vi "LSMcontroller_v60_PIzstage.vi"() -> ()   [LabVIEW 2015] (continued)
                                n1732 = Unbundle By Name(w4426) -> ("srate"=w4423:sgl, "Pel"=w4425:sgl)
                                n1733 = To Double Precision Float(number=w4423) -> (double precision float=w4421:dbl)
                                n1734 = To Double Precision Float(number=w4423) -> (double precision float=w4422:dbl)
                                n1735 = To Double Precision Float(number=w4425) -> (double precision float=w4417:dbl)
                                n1736 = Divide(x=w4422, y=w4417) -> (x/y=w4424:dbl)
                                n1737 = Index Array(array=w4434, index=0) -> (element=w4433:T19)
                                n1738 = Divide(x=1.0 ("Digital DC (%)"), y=w4417) -> (x/y=w4419:dbl)
                                n1739 = Multiply(x=100.0, y=w4419) -> (x*y=w4416:dbl)
                                n1740 = Bundle By Name(cluster=w4433, "Digital DC (%)"=w4416, "Digital phase"=w4428, "Digital Freq (Hz)"=w4424, "Sampling frequency (Hz)"=w4421, "Digital time offset (s)"=w4428, "padding value"=0.0, "matlab wave file"=path "LT", "DOtab"=0.0) -> (w4431:T19)
                                n1741 = Build Array(w4431) -> (w4430:T18)
                                n1742 = call "waveformparamsv2.vi"("command"="add DO", "add DO"=w4430) -> ()  [unwired: 3 in, 3 out]
                                }
                                frame 2 {
                                n1743 = call "waveformparamsv2.vi"("command"="get") -> ("Params out"=w4443:T15)  [unwired: 4 in, 2 out]
                                n1744 = in-place {
                                in-place-border: w4441 -> [w4447]
                                in-place-border: [w4446] -> w4440
                                n1745 = in-place-cluster #30(w4443) -> ("DO parameters"=w4449:T18)
                                n1746 = Delete From Array(array=w4449, length=1, index=w4447) -> (deleted portion=w4446:T18, array with subset deleted=w4448:T18)
                                n1747 = in-place-cluster #30("DO parameters"=w4448) -> (w4442:T15)
                                }
                                n1748 = call "waveformparamsv2.vi"("command"="set", "Params in"=w4442) -> ()  [unwired: 3 in, 3 out]
                                }
                                frame 3, Default {
                                }
                                frame 0 {
                                n1749 = local read "Measurement"() -> (w4455:T4)
                                n1750 = To Unsigned Long Integer(number=w4455) -> (unsigned 32bit integer=w4454:u32)
                                n1751 = case shown="5..7" w4454 {
                                tunnel: w4453 -> [_ w4457]
                                tunnel: [_ w4456] -> w4452
                                frame 0..4, Default {
                                }
                                frame 5..7 {
                                n1752 = stacked-sequence {
                                tunnel: w4457 -> [w4459 w4468]
                                tunnel: [w4458 _] -> w4456
                                frame #0 {
                                n1753 = call "waveformparamsv2.vi"("command"="get") -> ("Params out"=w4461:T15)  [unwired: 4 in, 2 out]
                                n1754 = Unbundle By Name(w4461) -> ("DO parameters"=w4462:T18)
                                n1755 = Index Array(array=w4462, index=w4459) -> (element=w4458:T19)
                                }
                                frame #1 {
                                w4476 = 0.0 ("padding value")
                                n1756 = call "2pparameters.vi"("command"="get") -> ("params out"=w4474:T11)  [unwired: 1 in]
                                n1757 = Unbundle By Name(w4474) -> ("srate"=w4472:sgl, "Pel"=w4473:sgl)
                                n1758 = To Double Precision Float(number=w4472) -> (double precision float=w4470:dbl)
                                n1759 = To Double Precision Float(number=w4472) -> (double precision float=w4471:dbl)
                                n1760 = To Double Precision Float(number=w4473) -> (double precision float=w4466:dbl)
                                n1761 = Divide(x=1.0 ("Digital DC (%)"), y=w4466) -> (x/y=w4465:dbl)
                                n1762 = Multiply(x=100.0, y=w4465) -> (x*y=w4464:dbl)
                                n1763 = Divide(x=w4471, y=w4466) -> (x/y=w4469:dbl)
                                n1764 = call "replace DO wf param.vi"("Digital Freq (Hz)"=w4469, "Digital DC (%)"=w4464, "Digital phase"=w4476, "Sampling frequency (Hz)"=w4470, "Digital time offset (s)"=w4476, "index of DO wave"=w4468, "padding value"=w4476, "matlab wave file"=path "LT" ("matlab wave number")) -> ()  [unwired: 3 in]
                                }
                                }
                                }
                                }
                                n1765 = Build Array(w4452) -> (w4451:T18)
                                }
                                }
                                }
                                frame #9 {
                                n1766 = Build Array(w4481, w4480) -> (w4483:bool[])
                                n1767 = Boolean Array To Number(Boolean array=w4483) -> (number=w4482:u32)
                                n1768 = case shown="0" w4482 {
                                tunnel: w4479 -> [_ w4535 _ w4539]
                                tunnel: [_ w4530 _ w4536] -> w4478
                                frame 1 {
                                n1769 = call "2pparameters.vi"("command"="get") -> ("params out"=w4490:T11)  [unwired: 1 in]
                                n1770 = Unbundle By Name(w4490) -> ("wavdet"=w4491:bool, "Pel"=w4493:sgl, "refwfsize"=w4494:dbl, "Pel"=w4492:sgl)
                                n1771 = call "waveformsDObuffer.vi"("command"="get") -> ("DO wf out"=w4486:digitalwaveform[])  [unwired: 1 in]
                                n1772 = case shown="True" w4491 {
                                tunnel: [w4498 w4511] -> w4488
                                tunnel: w4492 -> [w4507 w4526]
                                tunnel: w4493 -> [w4497 w4517]
                                tunnel: w4494 -> [_ w4523]
                                frame False {
                                w4501 = u16 0 items=["unsigned binary", "offset binary", "2's complement"] ("data format (offset binary)")
                                n1773 = Initialize Array(sgl 0.0, w4497) -> (w4504:sgl[])
                                n1774 = Replace Array Subset(array=w4504, new element=sgl 1.0, index=0) -> (w4502:sgl[])
                                n1775 = Reciprocal(x=w4507) -> (1/x=w4508:sgl)
                                n1776 = Bundle By Name("Y"=w4502, "dt"=w4508) -> (w4499:waveform(sgl))  [unwired: 1 in]
                                n1777 = call-poly <vilib>:"Analog to Digital.vi"("data format (offset binary)"=w4501, "compress digital (T)"=TRUE, "full-scale range (pk-pk)"=1.0, "resolution (16 bit)"=1, "analog waveform"=w4499) -> ("digital waveform"=w4498:digitalwaveform)  [unwired: 3 in, 3 out]
                                }
                                frame True {
                                w4514 = u16 0 items=["unsigned binary", "offset binary", "2's complement"] ("data format (offset binary)")
                                n1778 = To Double Precision Float(number=w4517) -> (double precision float=w4524:dbl)
                                n1779 = Initialize Array(sgl 0.0, w4517) -> (w4519:sgl[])
                                n1780 = Divide(x=w4523, y=w4524) -> (x/y=w4521:dbl)
                                n1781 = Round Toward +Infinity(x=w4521) -> (ceil(x): smallest int >= x=w4522:dbl)
                                n1782 = Replace Array Subset(array=w4519, new element=sgl 1.0, index=0) -> (w4516:sgl[])
                                n1783 = for {
                                N: w4522 -> [_]
                                tunnel: w4516 -> [w4528]
                                tunnel: [w4528] -> w4525 mode=concatenating
                                }
                                n1784 = Reciprocal(x=w4526) -> (1/x=w4527:sgl)
                                n1785 = Bundle By Name("Y"=w4525, "dt"=w4527) -> (w4512:waveform(sgl))  [unwired: 1 in]
                                n1786 = call-poly <vilib>:"Analog to Digital.vi"("data format (offset binary)"=w4514, "compress digital (T)"=TRUE, "full-scale range (pk-pk)"=1.0, "resolution (16 bit)"=1, "analog waveform"=w4512) -> ("digital waveform"=w4511:digitalwaveform)  [unwired: 3 in, 3 out]
                                }
                                }
                                n1787 = Build Array (concatenate)(w4486, w4488) -> (w4484:digitalwaveform[])
                                n1788 = call "waveformsDObuffer.vi"("DO wf in"=w4484, "command"="set") -> ()  [unwired: 1 out]
                                }
                                frame 2 {
                                n1789 = call "waveformsDObuffer.vi"("command"="get") -> ("DO wf out"=w4532:digitalwaveform[])  [unwired: 1 in]
                                n1790 = Delete From Array(array=w4532, length=1, index=w4535) -> (deleted portion=w4530:digitalwaveform[], array with subset deleted=w4529:digitalwaveform[])
                                n1791 = call "waveformsDObuffer.vi"("DO wf in"=w4529, "command"="set") -> ()  [unwired: 1 out]
                                }
                                frame 3, Default {
                                }
                                frame 0 {
                                n1792 = local read "Measurement"() -> (w4538:T4)
                                n1793 = To Unsigned Long Integer(number=w4538) -> (unsigned 32bit integer=w4537:u32)
                                n1794 = case shown="5..7" w4537 {
                                tunnel: w4539 -> [_ w4542]
                                tunnel: [_ w4541] -> w4536
                                frame 0..4, Default {
                                }
                                frame 5..7 {
                                n1795 = call "2pparameters.vi"("command"="get") -> ("params out"=w4549:T11)  [unwired: 1 in]
                                n1796 = Unbundle By Name(w4549) -> ("wavdet"=w4550:bool, "Pel"=w4552:sgl, "refwfsize"=w4553:dbl, "srateAODO"=w4551:sgl)
                                n1797 = call "waveformsDObuffer.vi"("command"="get") -> ("DO wf out"=w4543:digitalwaveform[])  [unwired: 1 in]
                                n1798 = Index Array(array=w4543, index=w4542) -> (element=w4544:digitalwaveform)
                                n1799 = case shown="True" w4550 {
                                tunnel: [w4557 w4570] -> w4547
                                tunnel: w4551 -> [w4566 w4585]
                                tunnel: w4552 -> [w4556 w4576]
                                tunnel: w4553 -> [_ w4582]
                                frame False {
                                w4560 = u16 0 items=["unsigned binary", "offset binary", "2's complement"] ("data format (offset binary)")
                                n1800 = Initialize Array(sgl 0.0, w4556) -> (w4563:sgl[])
                                n1801 = Replace Array Subset(array=w4563, new element=sgl 1.0, index=0) -> (w4561:sgl[])
                                n1802 = Reciprocal(x=w4566) -> (1/x=w4567:sgl)
                                n1803 = Bundle By Name("Y"=w4561, "dt"=w4567) -> (w4558:waveform(sgl))  [unwired: 1 in]
                                n1804 = call-poly <vilib>:"Analog to Digital.vi"("data format (offset binary)"=w4560, "compress digital (T)"=TRUE, "full-scale range (pk-pk)"=1.0, "resolution (16 bit)"=1, "analog waveform"=w4558) -> ("digital waveform"=w4557:digitalwaveform)  [unwired: 3 in, 3 out]
                                }
                                frame True {
                                w4573 = u16 0 items=["unsigned binary", "offset binary", "2's complement"] ("data format (offset binary)")
                                n1805 = To Double Precision Float(number=w4576) -> (double precision float=w4583:dbl)
                                n1806 = Initialize Array(sgl 0.0, w4576) -> (w4578:sgl[])
                                n1807 = Divide(x=w4582, y=w4583) -> (x/y=w4580:dbl)
                                n1808 = Round Toward +Infinity(x=w4580) -> (ceil(x): smallest int >= x=w4581:dbl)
                                n1809 = Replace Array Subset(array=w4578, new element=sgl 1.0, index=0) -> (w4575:sgl[])
                                n1810 = for {
                                N: w4581 -> [_]
                                tunnel: w4575 -> [w4587]
                                tunnel: [w4587] -> w4584 mode=concatenating
                                }
                                n1811 = Reciprocal(x=w4585) -> (1/x=w4586:sgl)
                                n1812 = Bundle By Name("Y"=w4584, "dt"=w4586) -> (w4571:waveform(sgl))  [unwired: 1 in]
                                n1813 = call-poly <vilib>:"Analog to Digital.vi"("data format (offset binary)"=w4573, "compress digital (T)"=TRUE, "full-scale range (pk-pk)"=1.0, "resolution (16 bit)"=1, "analog waveform"=w4571) -> ("digital waveform"=w4570:digitalwaveform)  [unwired: 3 in, 3 out]
                                }
                                }
                                n1814 = Build Array(w4544) -> (w4541:digitalwaveform[])
                                n1815 = Replace Array Subset(array=w4543, new element=w4547, index=w4542) -> (w4540:digitalwaveform[])
                                n1816 = call "waveformsDObuffer.vi"("DO wf in"=w4540, "command"="set") -> ()  [unwired: 1 out]
                                }
                                }
                                }
                                }
                                }
                                frame #10 {
                                n1817 = local read "Meastab"() -> (w4601:enum32{"X-Y Image", "Linescan", "Timetrace"})
                                n1818 = property on="refwf" class="Ring (strict)"() -> ("RingText.Text"=w4598:string)  [unwired: 2 in, 2 out]
                                n1819 = case shown="\"Timetrace\"" w4601 {
                                tunnel: [w4603 w4604] -> w4602
                                frame "X-Y Image", Default {
                                n1820 = local read "Sampling rate"() -> (w4603:dbl)
                                }
                                frame "Timetrace" {
                                n1821 = local read "srateAODOtt"() -> (w4604:dbl)
                                }
                                }
                                n1822 = call "waveformsAObuffer.vi"("command"="get") -> ("AO wf out"=w4591:waveform(dbl)[])  [unwired: 1 in]
                                n1823 = local read "wavdet"() -> (w4599:bool)
                                n1824 = call "waveformsDObuffer.vi"("command"="get") -> ("DO wf out"=w4595:digitalwaveform[])  [unwired: 1 in]
                                n1825 = call "correctwaveformsizetemp.vi"("new sampling frequency (Hz)"=w4602, "start"=TRUE, "reference waveforms to"=w4598, "Analog waveforms in"=w4591, "stop"=FALSE, "Digital waveforms in"=w4595) -> ("analog wf out"=w4597:waveform(dbl)[], "Digital wf out"=w4590:digitalwaveform[], "measpoints"=w4600:i32)
                                n1826 = call "waveformsDObuffer.vi"("DO wf in"=w4590, "command"="set") -> ()  [unwired: 1 out]
                                n1827 = call "waveformsAObuffer.vi"("AO wf in"=w4597, "command"="set") -> ()  [unwired: 1 out]
                                n1828 = case shown="True" w4599 {
                                tunnel: w4600 -> [_ w4607]
                                tunnel: w4590 -> [_ w4605]
                                frame False {
                                }
                                frame True {
                                n1829 = local write "# of frames"(w4607) -> ()
                                n1830 = call "GetNumCamFramesv2.vi"("Digital Waveform Graph"=w4605) -> ("Numeric"=w4606:i32)  [unwired: 10 in]
                                n1831 = local write "Total Camera Frames"(w4606) -> ()
                                }
                                }
                                }
                                }
                              }
                              frame #7 {
                                # "Disabled for conversion to 64 bit"
                                n1832 = disable-structure shown="Disabled" {
                                frame Disabled {
                                n1833 = local read "Measurement"() -> (w4609:T4)
                                n1834 = case shown="\"Lifetime (scan)\"" w4609 {
                                frame "X-Y-t movie", Default {
                                }
                                frame "Lifetime (scan)" {
                                # "total acquisition time"
                                n1835 = call "2pparameters.vi"("command"="get") -> ("params out"=w4617:T11)  [unwired: 1 in]
                                n1836 = Unbundle By Name(w4617) -> ("measpoints"=w4611:i32, "srateAODO"=w4632:sgl)
                                n1837 = Divide(x=w4611, y=w4632) -> (x/y=w4610:sgl)
                                n1838 = local read "min phot"() -> (w4627:u32)
                                n1839 = local read "expected c/s"() -> (w4628:dbl)
                                n1840 = Multiply(x=w4610, y=1000.0) -> (x*y=w4620:dbl)
                                n1841 = local read "Ch1 ZeroX"() -> (w4625:i32)
                                n1842 = local read "truncate"() -> (w4626:u32)
                                n1843 = To Long Integer(number=w4620) -> (32bit integer=w4629:i32)
                                n1844 = To Long Integer(number=w4628) -> (32bit integer=w4630:i32)
                                n1845 = local read "Number of Bins"() -> (w4621:u32)
                                n1846 = local read "Ch1 Level"() -> (w4623:i32)
                                n1847 = local read "Ch0 ZeroX"() -> (w4624:i32)
                                n1848 = local write "Acquisition time"(w4629) -> ()
                                n1849 = local read "Ch0 Level"() -> (w4622:i32)
                                n1850 = call "lifetimeparameters.vi"("command"="get") -> ("Params out"=w4615:T20)  [unwired: 1 in]
                                n1851 = Add(x=100, y=w4629) -> (x+y=w4619:i32)
                                n1852 = Bundle By Name(cluster=w4615, "acq time"=w4619, "acq rate"=w4630, "# bins"=w4621, "Ch0 Level"=w4622, "Ch1 Level"=w4623, "Ch0 ZeroX"=w4624, "Ch1 ZeroX"=w4625, "min photons"=w4627, "truncate"=w4626) -> (w4614:T20)
                                n1853 = local write "Acquisition rate"(w4630) -> ()
                                n1854 = call "lifetimeparameters.vi"("Params in"=w4614, "command"="set") -> ()  [unwired: 1 out]
                                }
                                }
                                }
                                frame Enabled {
                                }
                                }
                                n1855 = local write "64bit disabled"(TRUE ("64bit disabled")) -> ()
                              }
                              frame #8 {
                                n1856 = call "2pparameters.vi"("command"="get") -> ("params out"=w4643:T11)  [unwired: 1 in]
                                n1857 = Unbundle By Name(w4643) -> ("refreshbuffer"=w4641:i32, "srate"=w4642:sgl)
                                n1858 = local read "wavdet"() -> (w4633:bool)
                                n1859 = To Double Precision Float(number=w4642) -> (double precision float=w4645:dbl)
                                n1860 = To Double Precision Float(number=w4641) -> (double precision float=w4636:dbl)
                                n1861 = case shown="False" w4633 {
                                tunnel: [w4650 w4651] -> w4635
                                frame False {
                                w4650 = 10123 items=["Finite Samples"=10178, "Continuous Samples"=10123, "Hardware Timed Single Point"=12522] ("sample mode")
                                }
                                frame True {
                                w4651 = 10123 items=["Finite Samples"=10178, "Continuous Samples"=10123, "Hardware Timed Single Point"=12522] ("sample mode")
                                }
                                }
                                n1862 = Divide(x=w4636, y=w4645) -> (x/y=w4649:dbl)
                                n1863 = Multiply(x=w4649, y=2.0) -> (x*y=w4646:dbl)
                                n1864 = Max & Min(x=w4646, y=10.0) -> (max(x,y)=w4637:dbl)  [unwired: 1 out]
                                n1865 = call "2pparameters.vi"("command"="get") -> ("params out"=w4640:T11)  [unwired: 1 in]
                                n1866 = Bundle By Name(cluster=w4640, "timeout"=w4637, "sample mode"=w4635) -> (w4638:T11)
                                n1867 = call "2pparameters.vi"("Params in"=w4638, "command"="set") -> ()  [unwired: 1 out]
                              }
                            }
                          }
                          frame #1 {
                            # "Disabled for conversion to 64 bit"
                            n1868 = call "prepAO_img.vi"() -> ("Terminal Name with Device Prefix"=w4653:tag)
                            n1869 = call "prepDO_img.vi"() -> ()  [unwired: 2 in]
                            n1870 = call "prepAI_img.vi"("triggersource"=w4653) -> ()  [unwired: 2 in]
                            n1871 = call "prepCI_img.vi"("ArmStart.DigEdge.Src"=w4653) -> ()  [unwired: 1 in]
                            n1872 = disable-structure shown="Disabled" {
                              frame Disabled {
                                n1873 = local read "Measurement"() -> (w4654:T4)
                                n1874 = case shown="\"Lifetime (contour)\"" w4654 {
                                frame "X-Y-t movie", Default {
                                }
                                frame "Lifetime (contour)" {
                                n1875 = stacked-sequence {
                                frame #0 {
                                n1876 = call "PH-temp.vi"("String"="clear" ("command")) -> ()  [unwired: 2 in, 2 out]
                                n1877 = call "PH-temp-raw.vi"("command"="empty") -> ()  [unwired: 1 in, 1 out]
                                }
                                frame #1 {
                                n1878 = call "calib.vi"() -> ()  [unwired: 1 in]
                                }
                                frame #2 {
                                n1879 = call "setup.vi"() -> ()  [unwired: 1 in]
                                }
                                }
                                }
                                }
                              }
                              frame Enabled {
                              }
                            }
                            n1880 = local write "64bit disabled"(TRUE ("64bit disabled")) -> ()
                          }
                          frame #2 {
                            n1881 = local read "save\ndata"() -> (w4657:bool)
                            n1882 = case shown="True" w4657 {
                              tunnel: w4658 -> [_ w4662]
                              frame False {
                              }
                              frame True {
                                n1883 = local read "filename prefix"() -> (w4660:string)
                                n1884 = local read "data dir"() -> (w4661:path)
                                n1885 = call "preparebinaryfiles.vi"("filename prefix"=w4660, "data dir"=w4661, "timestamp"=w4662) -> ("full-filename"=w4659:string)  [unwired: 1 in]
                                n1886 = local write "full-filename"(w4659) -> ()
                              }
                            }
                            n1887 = call "preptempbuffers_tt.vi"() -> ()  [unwired: 12 in]
                          }
                          frame #3 {
                            n1888 = local read "wavdet"() -> (w4663:bool)
                            n1889 = case shown="False" w4663 {
                              frame False {
                                n1890 = disable-structure shown="Disabled" {
                                frame Disabled {
                                n1891 = call "2pparameters.vi"("command"="get") -> ("params out"=w4665:T11)  [unwired: 1 in]
                                n1892 = Unbundle By Name(w4665) -> ("autoshutter"=w4666:bool)
                                n1893 = case shown="True" w4666 {
                                frame False {
                                }
                                frame True {
                                n1894 = call "shuttercontrol.vi"("command"="open") -> ()  [unwired: 1 in, 1 out]
                                }
                                }
                                }
                                frame Enabled {
                                }
                                }
                              }
                              frame True {
                              }
                            }
                          }
                          frame #4 {
                            n1895 = flat-sequence {
                              frame #0 {
                                # "Disabled for conversion to 64 bit"
                                n1896 = disable-structure shown="Disabled" {
                                frame Disabled {
                                n1897 = local read "Measurement"() -> (w4669:T4)
                                n1898 = case shown="\"Lifetime (contour)\"" w4669 {
                                frame "X-Y-t movie", Default {
                                }
                                frame "Lifetime (contour)" {
                                n1899 = call "runLT_img.vi"() -> ()  [unwired: 1 in]
                                }
                                }
                                }
                                frame Enabled {
                                }
                                }
                                n1900 = local write "64bit disabled"(TRUE ("64bit disabled")) -> ()
                              }
                              frame #1 {
                                n1901 = call "runAI_img.vi"() -> ()  [unwired: 12 in]
                                n1902 = call "runCI.vi"() -> ()  [unwired: 12 in]
                                n1903 = call "runDO_img.vi"() -> ()  [unwired: 12 in]
                              }
                              frame #2 {
                                n1904 = call "runAO_img.vi"() -> ()  [unwired: 12 in]
                              }
                            }
                          }
                          frame #5 {
                            # "Disabled for conversion to 64 bit"
                            n1905 = disable-structure shown="Disabled" {
                              disable-tunnel: w4671 -> [w4672 _]
                              frame Disabled {
                                w4675 = u16 0 items=["Stream to disk", "Post process", "real time process"] ("Ring")
                                n1906 = local read "T3R Data processing"() -> (w4674:u16)
                                n1907 = Equal?(x=w4674, y=w4675) -> (x = y?=w4673:bool)
                                n1908 = local read "save\ndata"() -> (w4677:bool)
                                n1909 = local read "Measurement"() -> (w4678:T4)
                                n1910 = And(x=w4677, y=w4673) -> (x .and. y?=w4676:bool)
                                n1911 = case shown="\"Lifetime (contour)\"" w4678 {
                                tunnel: w4672 -> [_ w4682]
                                tunnel: w4676 -> [_ w4680]
                                frame "X-Y-t movie", Default {
                                }
                                frame "Lifetime (contour)" {
                                n1912 = case shown="True" w4680 {
                                selector: w4680 -> [w4683 w4688]
                                tunnel: w4682 -> [_ w4686]
                                tunnel: [path "" ("appended path") w4689] -> w4681
                                tunnel: [w4683 w4688] -> w4679
                                frame False {
                                }
                                frame True {
                                n1913 = local read "filename prefix"() -> (w4687:string)
                                n1914 = local read "data dir"() -> (w4690:path)
                                n1915 = call "generatedatafilename.vi"("timestamp"=w4686, "filename prefix in"=w4687) -> ("full-filename"=w4685:string)
                                n1916 = Concatenate Strings(w4685, ".lvpt3contour" ("string")) -> (w4692:string)
                                n1917 = Build Path(base path=w4690, name or relative path=w4692) -> (appended path=w4689:path)
                                }
                                }
                                n1918 = call "collectLT_res_v1.vi"("stream?"=w4679, "data file"=w4681) -> ()  [unwired: 2 out]
                                }
                                }
                              }
                              frame Enabled {
                              }
                            }
                            n1919 = while {
                              i -> [w4695]
                              stop <- w4693 stop-if-true
                              n1920 = local read "Stop"() -> (w4703:bool)
                              n1921 = local read "Exit"() -> (w4702:bool)
                              n1922 = Increment(x=w4695) -> (x+1=w4694:i32)
                              n1923 = local write "points recorded"(w4694) -> ()
                              n1924 = Or(x=w4703, y=w4702) -> (x .or. y?=w4701:bool)
                              n1925 = case shown="False" w4701 {
                                frame False {
                                n1926 = stacked-sequence {
                                frame #0 {
                                n1927 = call "collectAI_tt_V2.vi"() -> ()  [unwired: 4 in]
                                n1928 = call "collectCI_tt.vi"() -> ("size(s)"=w4710:i32)  [unwired: 3 in]
                                n1929 = local write "scol"(w4710) -> ()
                                }
                                frame #1 {
                                n1930 = local read "Live"() -> (w4711:bool)
                                n1931 = case shown="True" w4711 {
                                frame False {
                                }
                                frame True {
                                n1932 = local read "graph1list"() -> (w4718:u16)
                                n1933 = local read "graph2list"() -> (w4717:u16)
                                n1934 = To Unsigned Word Integer(number=w4718) -> (unsigned 16bit integer=w4716:u16)
                                n1935 = To Unsigned Word Integer(number=w4717) -> (unsigned 16bit integer=w4715:u16)
                                n1936 = call "dattotrace.vi"("graph2list"=w4715, "Current Average"=sgl 1.0, "graph1list"=w4716) -> ("trace2array out"=w4713:sgl[], "trace1array out"=w4724:sgl[])
                                n1937 = local read "bin"() -> (w4725:dbl)
                                n1938 = script code="data=reshape(datain,[bin length(datain)./bin]);\ndataout=mean(data,1);\ndata2=reshape(datain2,[bin length(datain2)./bin]);\ndataout2=mean(data2,1);"("bin"=w4725, "datain"=w4724, "datain2"=w4713) -> ("dataout"=w4723:dbl[], "dataout2"=w4712:dbl[])  [unwired: 1 in, 1 out]
                                n1939 = Array Size(array=w4712) -> (size(s)=w4726:i32)
                                n1940 = Divide(x=w4726, y=2) -> (x/y=w4728:dbl)
                                n1941 = Round To Nearest(number=w4728) -> (nearest integer value=w4730:dbl)
                                n1942 = Array Size(array=w4723) -> (size(s)=w4735:i32)
                                n1943 = Delete From Array(array=w4712, length=w4730, index=0) -> (deleted portion=w4721:dbl[], array with subset deleted=w4722:dbl[])
                                n1944 = Divide(x=w4735, y=2) -> (x/y=w4733:dbl)
                                n1945 = Round To Nearest(number=w4733) -> (nearest integer value=w4731:dbl)
                                n1946 = Delete From Array(array=w4723, length=w4731, index=0) -> (deleted portion=w4720:dbl[], array with subset deleted=w4719:dbl[])
                                n1947 = local write "graph2"(w4719) -> ()
                                n1948 = local write "graph1"(w4720) -> ()
                                n1949 = local write "graph3"(w4721) -> ()
                                n1950 = local write "graph4"(w4722) -> ()
                                }
                                }
                                }
                                frame #2 {
                                n1951 = local read "save\ndata"() -> (w4736:bool)
                                n1952 = case shown="True" w4736 {
                                frame False {
                                }
                                frame True {
                                n1953 = call "savebinaryfiles.vi"() -> ()  [unwired: 1 in]
                                }
                                }
                                }
                                }
                                }
                                frame True {
                                }
                              }
                              n1954 = local read "continuous"() -> (w4698:bool)
                              n1955 = case shown="False" w4698 {
                                tunnel: w4694 -> [w4708 _]
                                tunnel: [w4707 FALSE] -> w4696
                                frame False {
                                n1956 = call "2pparameters.vi"("command"="get") -> ("params out"=w4705:T11)  [unwired: 1 in]
                                n1957 = Unbundle By Name(w4705) -> ("tt_cycles"=w4704:i32)
                                n1958 = Greater Or Equal?(x=w4708, y=w4704) -> (x >= y?=w4707:bool)
                                }
                                frame True {
                                }
                              }
                              n1959 = local read "Stop"() -> (w4700:bool)
                              n1960 = local read "Exit"() -> (w4699:bool)
                              n1961 = Or(x=w4700, y=w4699) -> (x .or. y?=w4697:bool)
                              n1962 = Or(x=w4697, y=w4696) -> (x .or. y?=w4693:bool)
                            }
                            n1963 = local write "64bit disabled"(TRUE ("64bit disabled")) -> ()
                          }
                          frame #6 {
                            # "Disabled for conversion to 64 bit"
                            n1964 = local read "Measurement"() -> (w4739:T4)
                            n1965 = disable-structure shown="Disabled" {
                              disable-tunnel: w4739 -> [w4741 _]
                              disable-tunnel: w4738 -> [w4740 _]
                              frame Disabled {
                                n1966 = case shown="\"Lifetime (contour)\"" w4741 {
                                tunnel: w4740 -> [_ w4742]
                                frame "X-Y-t movie", Default {
                                }
                                frame "Lifetime (contour)" {
                                n1967 = stacked-sequence {
                                tunnel: w4742 -> [_ w4743]
                                frame #0 {
                                n1968 = flat-sequence {
                                frame #0 {
                                n1969 = call "stoperaseLT_img.vi"() -> ()  [unwired: 1 in]
                                }
                                }
                                }
                                frame #1 {
                                w4746 = u16 0 items=["Stream to disk", "Post process", "real time process"] ("Ring")
                                n1970 = local read "T3R Data processing"() -> (w4745:u16)
                                n1971 = local read "save\ndata"() -> (w4748:bool)
                                n1972 = Equal?(x=w4745, y=w4746) -> (x = y?=w4744:bool)
                                n1973 = Not(x=w4744) -> (.not. x?=w4749:bool)
                                n1974 = And(x=w4748, y=w4749) -> (x .and. y?=w4747:bool)
                                n1975 = case shown="True" w4747 {
                                tunnel: w4743 -> [_ w4750]
                                frame False {
                                }
                                frame True {
                                n1976 = local read "filename prefix"() -> (w4751:string)
                                n1977 = local read "data dir"() -> (w4767:path)
                                n1978 = call "2pparameters.vi"("command"="get") -> ("params out"=w4762:T11)  [unwired: 1 in]
                                n1979 = call "generatedatafilename.vi"("timestamp"=w4750, "filename prefix in"=w4751) -> ("full-filename"=w4752:string)
                                n1980 = Unbundle By Name(w4762) -> ("srate"=w4760:sgl, "Pel"=w4759:sgl, "measpoints"=w4757:i32)
                                n1981 = Concatenate Strings(w4752, ".lvpt3contour" ("string")) -> (w4765:string)
                                n1982 = Build Path(base path=w4767, name or relative path=w4765) -> (appended path=w4764:path)
                                n1983 = To Unsigned Long Integer(number=w4760) -> (unsigned 32bit integer=w4761:u32)
                                n1984 = To Unsigned Long Integer(number=w4759) -> (unsigned 32bit integer=w4758:u32)
                                n1985 = To Unsigned Long Integer(number=w4757) -> (unsigned 32bit integer=w4756:u32)
                                n1986 = call "PH-temp-raw.vi"("command"="get") -> ("array out"=w4755:u32[])  [unwired: 1 in]
                                n1987 = Build Array (concatenate)(w4761, w4758, w4756, w4755) -> (w4754:u32[])
                                n1988 = Open/Create/Replace File(file path (use dialog)=w4764, operation (0:open)=T8."replace or create") -> (refnum out=w4771:refnum<file>, error out=w4770:errorcluster)  [unwired: 4 in, 1 out]
                                n1989 = Write to Binary File(file (use dialog)=w4771, data=w4754, error in=w4770, 5:FALSE ("prepend array or string size? (T)")) -> (refnum out=w4768:refnum<file>, error out=w4769:errorcluster)  [unwired: 2 in, 1 out]
                                n1990 = Close File(refnum=w4768, error in=w4769) -> ()  [unwired: 2 out]
                                }
                                }
                                }
                                }
                                }
                                }
                              }
                              frame Enabled {
                              }
                            }
                            n1991 = local write "64bit disabled"(TRUE ("64bit disabled")) -> ()
                          }
                          frame #7 {
                            n1992 = call "reset AO_DO_v3.vi"() -> ()  [unwired: 12 in]
                          }
                          frame #8 {
                            n1993 = stacked-sequence {
                              tunnel: w4787 -> [w4790 _ _ _ _ _]
                              tunnel: w4784 -> [w4789 _ _ _ _ _]
                              tunnel: w4785 -> [w4788 _ _ _ _ _]
                              tunnel: w4786 -> [_ w4839 _ _ _ _]
                              tunnel: w4782 -> [_ w4838 w4893 w4990 _ _]
                              tunnel: w4783 -> [_ w4837 w4892 w4989 _ _]
                              tunnel: w4781 -> [_ _ _ w4988 _ _]
                              tunnel: w4780 -> [_ _ _ w4987 _ _]
                              tunnel: w4779 -> [_ _ w4890 _ _ _]
                              tunnel: w4778 -> [_ _ w4889 _ _ _]
                              tunnel: w4777 -> [_ _ w4887 _ _ _]
                              tunnel: w4776 -> [_ _ w4886 _ _ _]
                              tunnel: w4775 -> [_ _ _ w4985 _ _]
                              tunnel: w4774 -> [_ _ _ w4984 _ _]
                              frame #0 {
                                n1994 = case shown="False" w4790 {
                                tunnel: w4789 -> [_ w4812]
                                tunnel: w4788 -> [_ w4811]
                                frame True {
                                n1995 = stacked-sequence {
                                seq-local: [w4791 _ _] -> [_ w4803 w4808]
                                frame #0 {
                                n1996 = call "configuration.vi"("command"="get") -> ("config out"=w4797:T12)  [unwired: 2 in, 1 out]
                                n1997 = Unbundle By Name(w4797) -> ("Voltage to Xgalvo"=w4794:i32)
                                n1998 = call "2pparameters.vi"("command"="get") -> ("params out"=w4795:T11)  [unwired: 1 in]
                                n1999 = in-place {
                                in-place-border: w4794 -> [w4802]
                                in-place-border: [w4799] -> w4791
                                n2000 = in-place-cluster #31(w4795) -> ("aAO"=w4801:u32[])
                                n2001 = call "remove channel from active arrayv2.vi"("line array in"=w4801, "line to remove"=w4802) -> ("line array out"=w4800:u32[], "index"=w4799:i32)  [unwired: 1 out]
                                n2002 = in-place-cluster #31("aAO"=w4800) -> (w4792:T11)
                                }
                                n2003 = call "2pparameters.vi"("Params in"=w4792, "command"="set") -> ()  [unwired: 1 out]
                                }
                                frame #1 {
                                n2004 = call "waveformparamsv2.vi"("command"="rem AO", "index"=w4803) -> ()  [unwired: 3 in, 3 out]
                                }
                                frame #2 {
                                n2005 = call "waveformsAObuffer.vi"("command"="get") -> ("AO wf out"=w4809:waveform(dbl)[])  [unwired: 1 in]
                                n2006 = Delete From Array(array=w4809, length=1, index=w4808) -> (array with subset deleted=w4805:waveform(dbl)[])  [unwired: 1 out]
                                n2007 = call "waveformsAObuffer.vi"("AO wf in"=w4805, "command"="set") -> ()  [unwired: 1 out]
                                }
                                }
                                }
                                frame False {
                                n2008 = stacked-sequence {
                                seq-local: [w4813 _ _] -> [_ w4821 w4832]
                                tunnel: w4812 -> [_ w4820 _]
                                tunnel: w4811 -> [_ _ w4831]
                                frame #0 {
                                n2009 = call "configuration.vi"("command"="get") -> ("config out"=w4818:T12)  [unwired: 2 in, 1 out]
                                n2010 = Unbundle By Name(w4818) -> ("Voltage to Xgalvo"=w4814:i32)
                                n2011 = call "2pparameters.vi"("command"="get") -> ("params out"=w4817:T11)  [unwired: 1 in]
                                n2012 = Unbundle By Name(w4817) -> ("aAO"=w4815:u32[])
                                n2013 = Search 1D Array(1D array=w4815, element=w4814) -> (index of element=w4813:i32)  [unwired: 1 in]
                                }
                                frame #1 {
                                n2014 = call "waveformparamsv2.vi"("command"="get") -> ("Params out"=w4824:T15)  [unwired: 4 in, 2 out]
                                n2015 = in-place {
                                in-place-border: w4821 -> [w4828]
                                in-place-border: w4820 -> [w4827]
                                n2016 = in-place-cluster #32(w4824) -> ("AO parameters"=w4829:T16)
                                n2017 = in-place {
                                in-place-border: w4827 -> [w4830]
                                n2018 = in-place-array #33(w4829, w4828) -> ()  [unwired: 1 out]
                                n2019 = in-place-array #33(w4830) -> (w4826:T16)  [unwired: 1 out]
                                }
                                n2020 = in-place-cluster #32("AO parameters"=w4826) -> (w4822:T15)
                                }
                                n2021 = call "waveformparamsv2.vi"("command"="set", "Params in"=w4822) -> ()  [unwired: 3 in, 3 out]
                                }
                                frame #2 {
                                n2022 = call "waveformsAObuffer.vi"("command"="get") -> ("AO wf out"=w4835:waveform(dbl)[])  [unwired: 1 in]
                                n2023 = Replace Array Subset(array=w4835, new element=w4831, index=w4832) -> (w4833:waveform(dbl)[])
                                n2024 = call "waveformsAObuffer.vi"("AO wf in"=w4833, "command"="set") -> ()  [unwired: 1 out]
                                }
                                }
                                }
                                }
                              }
                              frame #1 {
                                n2025 = case shown="False" w4839 {
                                tunnel: w4838 -> [_ w4861]
                                tunnel: w4837 -> [_ w4860]
                                frame True {
                                n2026 = stacked-sequence {
                                seq-local: [w4840 _ _] -> [_ w4852 w4857]
                                frame #0 {
                                n2027 = call "configuration.vi"("command"="get") -> ("config out"=w4846:T12)  [unwired: 2 in, 1 out]
                                n2028 = Unbundle By Name(w4846) -> ("Voltage to Ygalvo"=w4843:i32)
                                n2029 = call "2pparameters.vi"("command"="get") -> ("params out"=w4844:T11)  [unwired: 1 in]
                                n2030 = in-place {
                                in-place-border: w4843 -> [w4851]
                                in-place-border: [w4848] -> w4840
                                n2031 = in-place-cluster #34(w4844) -> ("aAO"=w4850:u32[])
                                n2032 = call "remove channel from active arrayv2.vi"("line array in"=w4850, "line to remove"=w4851) -> ("line array out"=w4849:u32[], "index"=w4848:i32)  [unwired: 1 out]
                                n2033 = in-place-cluster #34("aAO"=w4849) -> (w4841:T11)
                                }
                                n2034 = call "2pparameters.vi"("Params in"=w4841, "command"="set") -> ()  [unwired: 1 out]
                                }
                                frame #1 {
                                n2035 = call "waveformparamsv2.vi"("command"="rem AO", "index"=w4852) -> ()  [unwired: 3 in, 3 out]
                                }
                                frame #2 {
                                n2036 = call "waveformsAObuffer.vi"("command"="get") -> ("AO wf out"=w4858:waveform(dbl)[])  [unwired: 1 in]
                                n2037 = Delete From Array(array=w4858, length=1, index=w4857) -> (array with subset deleted=w4854:waveform(dbl)[])  [unwired: 1 out]
                                n2038 = call "waveformsAObuffer.vi"("AO wf in"=w4854, "command"="set") -> ()  [unwired: 1 out]
                                }
                                }
                                }
                                frame False {
                                n2039 = stacked-sequence {
                                seq-local: [w4862 _ _] -> [_ w4870 w4881]
                                tunnel: w4861 -> [_ w4869 _]
                                tunnel: w4860 -> [_ _ w4880]
                                frame #0 {
                                n2040 = call "configuration.vi"("command"="get") -> ("config out"=w4867:T12)  [unwired: 2 in, 1 out]
                                n2041 = Unbundle By Name(w4867) -> ("Voltage to Ygalvo"=w4863:i32)
                                n2042 = call "2pparameters.vi"("command"="get") -> ("params out"=w4866:T11)  [unwired: 1 in]
                                n2043 = Unbundle By Name(w4866) -> ("aAO"=w4864:u32[])
                                n2044 = Search 1D Array(1D array=w4864, element=w4863) -> (index of element=w4862:i32)  [unwired: 1 in]
                                }
                                frame #1 {
                                n2045 = call "waveformparamsv2.vi"("command"="get") -> ("Params out"=w4873:T15)  [unwired: 4 in, 2 out]
                                n2046 = in-place {
                                in-place-border: w4870 -> [w4877]
                                in-place-border: w4869 -> [w4876]
                                n2047 = in-place-cluster #35(w4873) -> ("AO parameters"=w4878:T16)
                                n2048 = in-place {
                                in-place-border: w4876 -> [w4879]
                                n2049 = in-place-array #36(w4878, w4877) -> ()  [unwired: 1 out]
                                n2050 = in-place-array #36(w4879) -> (w4875:T16)  [unwired: 1 out]
                                }
                                n2051 = in-place-cluster #35("AO parameters"=w4875) -> (w4871:T15)
                                }
                                n2052 = call "waveformparamsv2.vi"("command"="set", "Params in"=w4871) -> ()  [unwired: 3 in, 3 out]
                                }
                                frame #2 {
                                n2053 = call "waveformsAObuffer.vi"("command"="get") -> ("AO wf out"=w4884:waveform(dbl)[])  [unwired: 1 in]
                                n2054 = Replace Array Subset(array=w4884, new element=w4880, index=w4881) -> (w4882:waveform(dbl)[])
                                n2055 = call "waveformsAObuffer.vi"("AO wf in"=w4882, "command"="set") -> ()  [unwired: 1 out]
                                }
                                }
                                }
                                }
                              }
                              frame #2 {
                                n2056 = Build Array(w4890, w4889) -> (w4891:bool[])
                                n2057 = Boolean Array To Number(Boolean array=w4891) -> (number=w4888:u32)
                                n2058 = case shown="2" w4888 {
                                tunnel: w4893 -> [_ _ w4936]
                                tunnel: w4892 -> [_ _ w4935]
                                tunnel: w4887 -> [_ w4915 w4934]
                                tunnel: w4886 -> [_ w4914 w4933]
                                frame 1, Default {
                                n2059 = stacked-sequence {
                                seq-local: [w4894 _ _] -> [_ w4906 w4911]
                                frame #0 {
                                n2060 = call "configuration.vi"("command"="get") -> ("config out"=w4900:T12)  [unwired: 2 in, 1 out]
                                n2061 = Unbundle By Name(w4900) -> ("2P shutter"=w4897:i32)
                                n2062 = call "2pparameters.vi"("command"="get") -> ("params out"=w4898:T11)  [unwired: 1 in]
                                n2063 = in-place {
                                in-place-border: w4897 -> [w4905]
                                in-place-border: [w4902] -> w4894
                                n2064 = in-place-cluster #37(w4898) -> ("aDO"=w4904:u32[])
                                n2065 = call "remove channel from active arrayv2.vi"("line array in"=w4904, "line to remove"=w4905) -> ("line array out"=w4903:u32[], "index"=w4902:i32)  [unwired: 1 out]
                                n2066 = in-place-cluster #37("aDO"=w4903) -> (w4895:T11)
                                }
                                n2067 = call "2pparameters.vi"("Params in"=w4895, "command"="set") -> ()  [unwired: 1 out]
                                }
                                frame #1 {
                                n2068 = call "waveformparamsv2.vi"("command"="rem DO", "index"=w4906) -> ()  [unwired: 3 in, 3 out]
                                }
                                frame #2 {
                                n2069 = call "waveformsDObuffer.vi"("command"="get") -> ("DO wf out"=w4912:digitalwaveform[])  [unwired: 1 in]
                                n2070 = Delete From Array(array=w4912, length=1, index=w4911) -> (array with subset deleted=w4908:digitalwaveform[])  [unwired: 1 out]
                                n2071 = call "waveformsDObuffer.vi"("DO wf in"=w4908, "command"="set") -> ()  [unwired: 1 out]
                                }
                                }
                                }
                                frame 2 {
                                n2072 = stacked-sequence {
                                tunnel: w4915 -> [_ w4926 _]
                                tunnel: w4914 -> [_ _ w4928]
                                frame #0 {
                                n2073 = call "configuration.vi"("command"="get") -> ("config out"=w4917:T12)  [unwired: 2 in, 1 out]
                                n2074 = call "2pparameters.vi"("command"="get") -> ("params out"=w4921:T11)  [unwired: 1 in]
                                n2075 = Unbundle By Name(w4917) -> ("2P shutter"=w4916:i32)
                                n2076 = in-place {
                                in-place-border: w4916 -> [w4925]
                                n2077 = in-place-cluster #38(w4921) -> ("aDO"=w4924:u32[])
                                n2078 = call "add channel to active arrayv2.vi"("line array in"=w4924, "line to add"=w4925) -> ("line array out"=w4923:u32[])  [unwired: 2 out]
                                n2079 = in-place-cluster #38("aDO"=w4923) -> (w4919:T11)
                                }
                                n2080 = call "2pparameters.vi"("Params in"=w4919, "command"="set") -> ()  [unwired: 1 out]
                                }
                                frame #1 {
                                n2081 = call "waveformparamsv2.vi"("command"="add DO", "add DO"=w4926) -> ()  [unwired: 3 in, 3 out]
                                }
                                frame #2 {
                                n2082 = call "waveformsDObuffer.vi"("command"="get") -> ("DO wf out"=w4931:digitalwaveform[])  [unwired: 1 in]
                                n2083 = Build Array (concatenate)(w4931, w4928) -> (w4930:digitalwaveform[])
                                n2084 = call "waveformsDObuffer.vi"("DO wf in"=w4930, "command"="set") -> ()  [unwired: 1 out]
                                }
                                }
                                }
                                frame 0 {
                                n2085 = stacked-sequence {
                                seq-local: [w4937 _ _] -> [_ w4945 w4967]
                                tunnel: w4936 -> [_ _ _]
                                tunnel: w4935 -> [_ _ _]
                                tunnel: w4934 -> [_ w4944 _]
                                tunnel: w4933 -> [_ _ w4966]
                                frame #0 {
                                n2086 = call "configuration.vi"("command"="get") -> ("config out"=w4942:T12)  [unwired: 2 in, 1 out]
                                n2087 = call "2pparameters.vi"("command"="get") -> ("params out"=w4941:T11)  [unwired: 1 in]
                                n2088 = Unbundle By Name(w4942) -> ("2P shutter"=w4938:i32)
                                n2089 = Unbundle By Name(w4941) -> ("aDO"=w4939:u32[])
                                n2090 = Search 1D Array(1D array=w4939, element=w4938) -> (index of element=w4937:i32)  [unwired: 1 in]
                                }
                                frame #1 {
                                n2091 = call "2pparameters.vi"("command"="get") -> ("params out"=w4948:T11)  [unwired: 1 in]
                                n2092 = Unbundle By Name(w4948) -> ("wavdet"=w4946:bool, "autoshutter"=w4947:bool)
                                n2093 = case shown="True" w4947 {
                                tunnel: w4945 -> [_ w4952]
                                tunnel: w4946 -> [_ w4951]
                                tunnel: w4944 -> [_ w4950]
                                frame False {
                                }
                                frame True {
                                n2094 = case shown="False" w4951 {
                                tunnel: w4952 -> [w4956 _]
                                tunnel: w4950 -> [w4953 _]
                                frame False {
                                n2095 = Index Array(array=w4953, index=0) -> (element=w4954:T19)
                                n2096 = call "waveformparamsv2.vi"("command"="get") -> ("Params out"=w4959:T15)  [unwired: 4 in, 2 out]
                                n2097 = in-place {
                                in-place-border: w4956 -> [w4963]
                                in-place-border: w4954 -> [w4961]
                                n2098 = in-place-cluster #39(w4959) -> ("DO parameters"=w4964:T18)
                                n2099 = in-place {
                                in-place-border: w4961 -> [w4965]
                                n2100 = in-place-array #40(w4964, w4963) -> ()  [unwired: 1 out]
                                n2101 = in-place-array #40(w4965) -> (w4962:T18)  [unwired: 1 out]
                                }
                                n2102 = in-place-cluster #39("DO parameters"=w4962) -> (w4957:T15)
                                }
                                n2103 = call "waveformparamsv2.vi"("command"="set", "Params in"=w4957) -> ()  [unwired: 3 in, 3 out]
                                }
                                frame True {
                                }
                                }
                                }
                                }
                                }
                                frame #2 {
                                n2104 = call "2pparameters.vi"("command"="get") -> ("params out"=w4970:T11)  [unwired: 1 in]
                                n2105 = Unbundle By Name(w4970) -> ("wavdet"=w4968:bool, "autoshutter"=w4969:bool)
                                n2106 = case shown="True" w4969 {
                                tunnel: w4967 -> [_ w4974]
                                tunnel: w4968 -> [_ w4973]
                                tunnel: w4966 -> [_ w4972]
                                frame False {
                                }
                                frame True {
                                n2107 = case shown="False" w4973 {
                                tunnel: w4974 -> [w4978 _]
                                tunnel: w4972 -> [w4976 _]
                                frame False {
                                n2108 = Index Array(array=w4976, index=0) -> (element=w4975:digitalwaveform)
                                n2109 = call "waveformsDObuffer.vi"("command"="get") -> ("DO wf out"=w4980:digitalwaveform[])  [unwired: 1 in]
                                n2110 = Replace Array Subset(array=w4980, new element=w4975, index=w4978) -> (w4982:digitalwaveform[])
                                n2111 = call "waveformsDObuffer.vi"("DO wf in"=w4982, "command"="set") -> ()  [unwired: 1 out]
                                }
                                frame True {
                                }
                                }
                                }
                                }
                                }
                                }
                                }
                                }
                              }
                              frame #3 {
                                n2112 = Build Array(w4985, w4984) -> (w4986:bool[])
                                n2113 = Boolean Array To Number(Boolean array=w4986) -> (number=w4983:u32)
                                n2114 = case shown="2" w4983 {
                                tunnel: w4990 -> [_ _ w5033]
                                tunnel: w4989 -> [_ _ w5032]
                                tunnel: w4988 -> [_ w5012 w5030]
                                tunnel: w4987 -> [_ w5011 w5031]
                                frame 1, Default {
                                n2115 = stacked-sequence {
                                seq-local: [w4991 _ _] -> [_ w5003 w5008]
                                frame #0 {
                                n2116 = call "configuration.vi"("command"="get") -> ("config out"=w4997:T12)  [unwired: 2 in, 1 out]
                                n2117 = Unbundle By Name(w4997) -> ("LT timestamp"=w4994:u32)
                                n2118 = call "2pparameters.vi"("command"="get") -> ("params out"=w4995:T11)  [unwired: 1 in]
                                n2119 = in-place {
                                in-place-border: w4994 -> [w5002]
                                in-place-border: [w4999] -> w4991
                                n2120 = in-place-cluster #41(w4995) -> ("aDO"=w5001:u32[])
                                n2121 = call "remove channel from active arrayv2.vi"("line array in"=w5001, "line to remove"=w5002) -> ("line array out"=w5000:u32[], "index"=w4999:i32)  [unwired: 1 out]
                                n2122 = in-place-cluster #41("aDO"=w5000) -> (w4992:T11)
                                }
                                n2123 = call "2pparameters.vi"("Params in"=w4992, "command"="set") -> ()  [unwired: 1 out]
                                }
                                frame #1 {
                                n2124 = call "waveformparamsv2.vi"("command"="rem DO", "index"=w5003) -> ()  [unwired: 3 in, 3 out]
                                }
                                frame #2 {
                                n2125 = call "waveformsDObuffer.vi"("command"="get") -> ("DO wf out"=w5009:digitalwaveform[])  [unwired: 1 in]
                                n2126 = Delete From Array(array=w5009, length=1, index=w5008) -> (array with subset deleted=w5005:digitalwaveform[])  [unwired: 1 out]
                                n2127 = call "waveformsDObuffer.vi"("DO wf in"=w5005, "command"="set") -> ()  [unwired: 1 out]
                                }
                                }
                                }
                                frame 2 {
                                n2128 = stacked-sequence {
                                tunnel: w5012 -> [_ _ w5025]
                                tunnel: w5011 -> [_ w5023 _]
                                frame #0 {
                                n2129 = call "configuration.vi"("command"="get") -> ("config out"=w5014:T12)  [unwired: 2 in, 1 out]
